vi "brownian_motion.vi"() -> ()   [LabVIEW 2023]
panel:
  out "Walk":cluster{dbl[], dbl[]}(graph)
  out "i":i32
  in  "stop":bool
  in  "N":i32
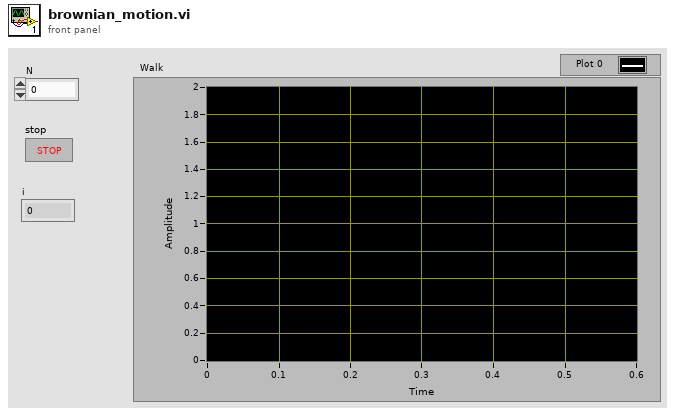
[diagram p1: front panel]
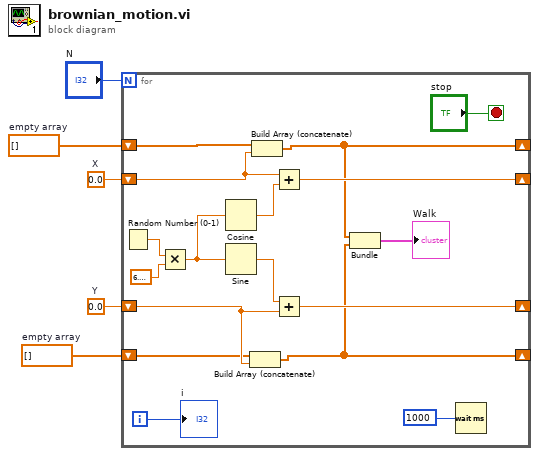
[diagram p0: block diagram]
diagram:
  w1 = dbl[] []  # empty array
  w2 = 0.0  # Y
  w3 = dbl[] []  # empty array
  w4 = 0.0  # X
  n1 = for {
    N: "N" -> [_]
    shift-right: [w10] -> _
    shift-left: w4 -> [w21]
    shift-right: [w9] -> _
    shift-left: w3 -> [w22]
    shift-right: [w11] -> _
    shift-left: w2 -> [w13]
    shift-right: [w8] -> _
    shift-left: w1 -> [w12]
    i -> [w16]
    stop <- "stop" stop-if-true
    n2 = Random Number (0-1)() -> (number: 0 to 1=w19:dbl)
    n3 = Multiply(x=w19, y=6.283185307179586) -> (x*y=w20:dbl)
    n4 = Cosine(x=w20) -> (cos(x)=w17:dbl)
    n5 = Sine(x=w20) -> (sin(x)=w14:dbl)
    n6 = Build Array (concatenate)(w12, w13) -> (w8:dbl[])
    n7 = Build Array (concatenate)(w22, w21) -> (w9:dbl[])
    n8 = Add(x=w21, y=w17) -> (x+y=w10:dbl)
    n9 = Add(x=w14, y=w13) -> (x+y=w11:dbl)
    n10 = Bundle(w9, w8) -> (→"Walk":cluster{dbl[], dbl[]})  [unwired: 1 in]
    n11 = Wait (ms)(milliseconds to wait=1000) -> ()  [unwired: 1 out]
    "i" <- w16
  }
